vi "init.vi"(2 "error in":errorcluster, 3 "Password":string="1234", 4 "User Name":string="git", 5 "Host Address":string="10.13.7.56") -> (0 "error out":errorcluster, 1 "prompt before $ sign":string)   [LabVIEW 2016, in "labssh_thijs.lvlib"]
uses:
  labssh_thijs.lvlib
  Labview SSH driver/state machine.ctl
  Labview SSH driver/store retrieve.ctl
panel:
  out "output one cr":string
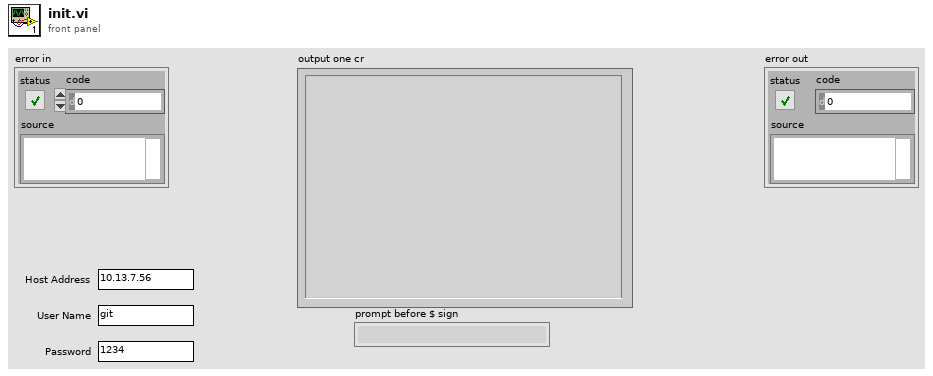
[diagram p1: front panel]
types:
  T1 = typedef "labssh_thijs.lvlib/store retrieve.ctl" = enum16{"store", "retrieve"}
  T2 = typedef "labssh_thijs.lvlib/state machine.ctl" = enum16{"init", "connect", "execute", "close", "exit", "read"}
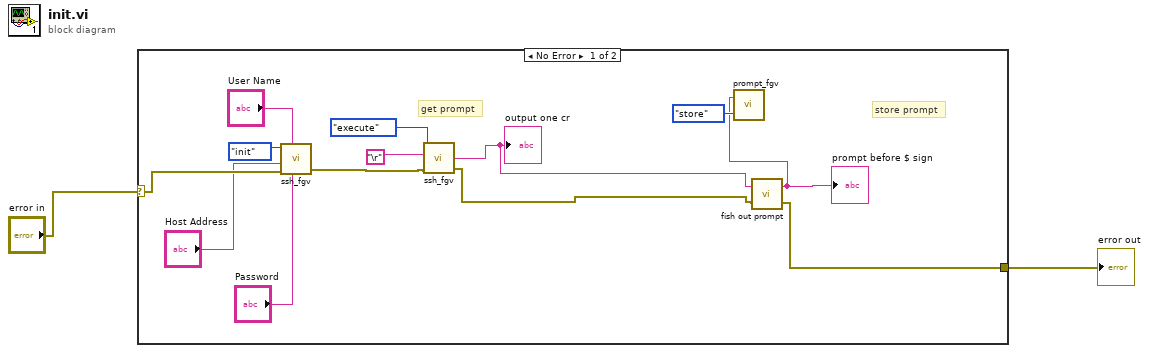
[diagram p0: block diagram]
diagram:
  n1 = case shown="No Error" "error in" {
    selector: "error in" -> [w14 w16]
    tunnel: [w8 w16] -> w1
    frame No Error {
      # "store prompt"
      # "get prompt"
      n2 = call "ssh_fgv.vi"(0:state_machine."init", "User Name"="User Name", "Host Address"="Host Address", "Password"="Password", "error in"=w14) -> ("error out"=w11:errorcluster)  [unwired: 2 in, 1 out]
      n3 = call "ssh_fgv.vi"(0:state_machine."execute", "Input"="\r", "error in"=w11) -> ("output_new"=w10:string, "error out"=w9:errorcluster)  [unwired: 4 in]
      "output one cr" <- w10
      n4 = call "fish out prompt.vi"("error in"=w9, "input string"=w10) -> ("error out"=w8:errorcluster, "prompt before $ sign"=w6:string)
      "prompt before $ sign" <- w6
      n5 = call "prompt_fgv.vi"(1:store_retrieve."store", "String in"=w6) -> ()  [unwired: 1 out]
    }
    frame Error {
    }
  }
  "error out" <- w1
